vi "AddSubscriber.vi"(8 "ErrorIn":errorcluster, 9 "Filters":T1[](array[typedef]), 11 "TAFTraceWindowIn":refnum<class "TAFTraceWindow.lvclass">) -> (0 "ErrorOut":errorcluster, 1 "TraceQueue":refnum<queue>, 3 "TAFTraceWindowOut":refnum<class "TAFTraceWindow.lvclass">)   [LabVIEW 2021, in "TAFTraceWindow.lvclass"]
uses:
  TAFTraceWindow.lvclass
  C:/Localdata/Projects/TriekselSoft/TriekselsoftApplicationFramework/Source/.Externals/Library_TAF/YActor/YActor.lvclass
  FilterConfiguration.ctl
  FilterFunction.ctl
  Library_TAF/YActor/YActor.lvclass/YActor.ctl
  Library_TAF/YActor/ExeCmd_sync.vi
  7918b6d0-a6dc-4851-a0dd-3936579228db.vi
  Library_TAF/YActor/private/SendCommand.vi
  Library_TAF/YActor/private/WaitForReply.vi
  Library_TAF/YActor/private/CreateLocalVI.vi
  Library_TAF/YActor/private/ExeuteInlineVI.vi
  Library_TAF/YActor/private/GetRemoteVIRef.vi
  Library_TAF/YActor/private/GetNameOfVI.vi
  Library_TAF/YActor/QuickCast.vi
  Library_TAF/YActor/private/VINameProperty.vi
  Library_TAF/YActor/private/MessageCounter.vi
  Library_TAF/YActor/InlineReferencePool.vi
  Library_TAF/YActor/private/ExecuteVI.vi
  Library_TAF/YActor/YActor.lvclass
  C:/Localdata/Projects/TriekselSoft/TriekselsoftApplicationFramework/Source/.Externals/Library_TAF/YAFTAF/YAFTAF.lvclass
  C:/Localdata/Projects/TriekselSoft/TriekselsoftApplicationFramework/Source/.Externals/Interface_UserInterface_IFrontPanel/IFrontPanel/IFrontPanel.lvclass
  C:/Localdata/Projects/TriekselSoft/TriekselsoftApplicationFramework/Source/.Externals/Interface_TAF_IInterface/IInterface/IInterface.lvclass
  C:/Localdata/Projects/TriekselSoft/TriekselsoftApplicationFramework/Source/.Externals/Interface_Object_ICreateDestroy/ICreateDestroy/ICreateDestroy.lvclass
  C:/Localdata/Projects/TriekselSoft/TriekselsoftApplicationFramework/Source/.Externals/Interface_Object_IPersistentData/IPersistentData/IPersistentData.lvclass
  C:/Localdata/Projects/TriekselSoft/TriekselsoftApplicationFramework/Source/.Externals/Interface_TAF_ITAFObject/ITAFObject/ITAFObject.lvclass
  C:/Localdata/Projects/TriekselSoft/TriekselsoftApplicationFramework/Source/.Externals/Library_TAF_TraceWindow/TAFTraceWindow/TAFTraceWindow.lvclass
  C:/Localdata/Projects/TriekselSoft/TriekselsoftApplicationFramework/Source/.Externals/Interface_TAF_TraceSubscriptor/ITAFFilteredTrace/ITAFFilteredTrace.lvclass
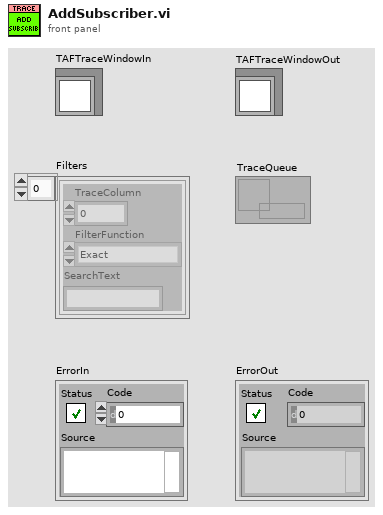
[diagram p1: front panel]
types:
  T1 = typedef "TAFTraceWindow.lvclass/FilterConfiguration.ctl" = cluster{"TraceColumn":i32, "FilterFunction":T2, "SearchText":string}
  T2 = typedef "TAFTraceWindow.lvclass/FilterFunction.ctl" = enum16{"Exact", "Regex"}
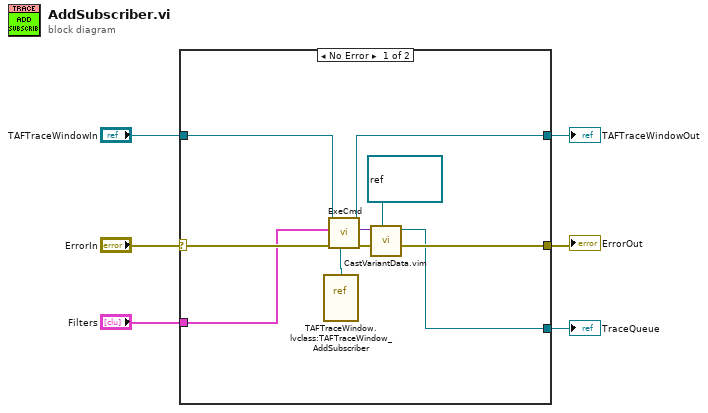
[diagram p0: block diagram]
diagram:
  n1 = case shown="No Error" "ErrorIn" {
    selector: "ErrorIn" -> [w16 w18]
    tunnel: [w14 w18] -> w5
    tunnel: [w10 w17] -> w3
    tunnel: "TAFTraceWindowIn" -> [w11 w17]
    tunnel: [w9 _] -> w2
    tunnel: "Filters" -> [w8 _]
    frame No Error {
      n2 = vi-ref "TAFTraceWindow.lvclass:TAFTraceWindow_AddSubscriber.vi"() -> (w13:refnum<vi>)
      n3 = call-poly "ExeCmd.vi"("CmdVIRef"=w13, "ErrorIn"=w16, "CmdData"=w8, "YActorIn"=w11) -> ("ErrorOut"=w15:errorcluster, "ReplyData"=w12:variant, "YActorOut"=w10:refnum<class "TAFTraceWindow.lvclass">)  [unwired: 5 in]
      n4 = call "CastVariantData.vim"("Type"=refnum<queue> refnum ("queue out"), "ErrorIn"=w15, "DataIn"=w12) -> ("ErrorOut"=w14:errorcluster, "DataOut"=w9:refnum<queue>)  [unwired: 7 in]
    }
    frame Error {
    }
  }
  "ErrorOut" <- w5
  "TAFTraceWindowOut" <- w3
  "TraceQueue" <- w2
